vi "Launch.vi"() -> ()   [LabVIEW 2020]
uses:
  Supervision/Supervision/Supervision.lvclass
  D:/Projets/STEP AT/LUGE 2022.2/UIA_Demo/support/UI_Actor.lvlibp/UI_Actor/UI_Actor.lvclass
  D&Cs/SCHEMA_01/SCHEMA_01/SCHEMA_01.lvclass
  D&Cs/SCHEMA_02/SCHEMA_02/SCHEMA_02.lvclass
  D&Cs/SCHEMA_03/SCHEMA_03/SCHEMA_03.lvclass
  support/UI_Actor.lvlibp/UI_Actor/ctl_AR_Parameters.ctl
  support/UI_Actor.lvlibp/UI_Actor/ctl_AR_Mode.ctl
  support/UI_Actor.lvlibp/UI_Actor/UI_Actor.lvclass
  support/UI_Actor.lvlibp/UI_Actor Messages/UI_AutoRefresh Msg/UI_AutoRefresh Msg.lvclass
  support/Databox.lvlibp
panel:
  in  "T_0":dbl(slide)=6.037735849056604 scale=0.0..10.0
  # "UIA Demo"
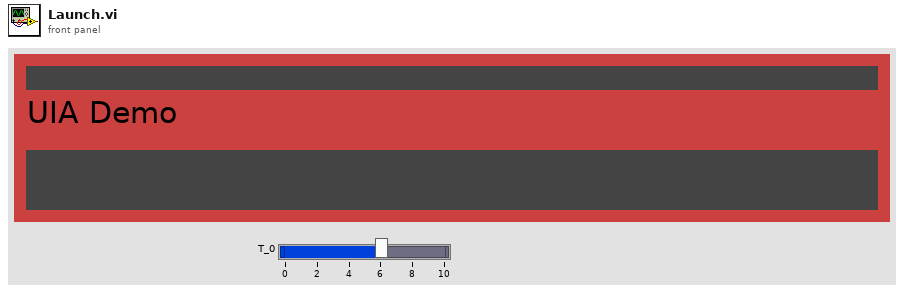
[diagram p1: front panel]
types:
  T1 = typedef "UI_Actor.lvlibp/UI_Actor.lvclass/ctl_AR_Parameters.ctl" = cluster{"Write TipStrips with details (T)":bool, "Write Captions with UserLabels (T)":bool, "Mode (ind only)":T2, "Enable nested stream (T)":bool}
  T2 = typedef "UI_Actor.lvlibp/UI_Actor.lvclass/ctl_AR_Mode.ctl" = enum16{"Controls only", "Indicators only", "All"}
  T3 = cluster{"Ch.Conf":refnum<class "Config.lvclass">, "Data":refnum<class "Data.lvclass">[]}
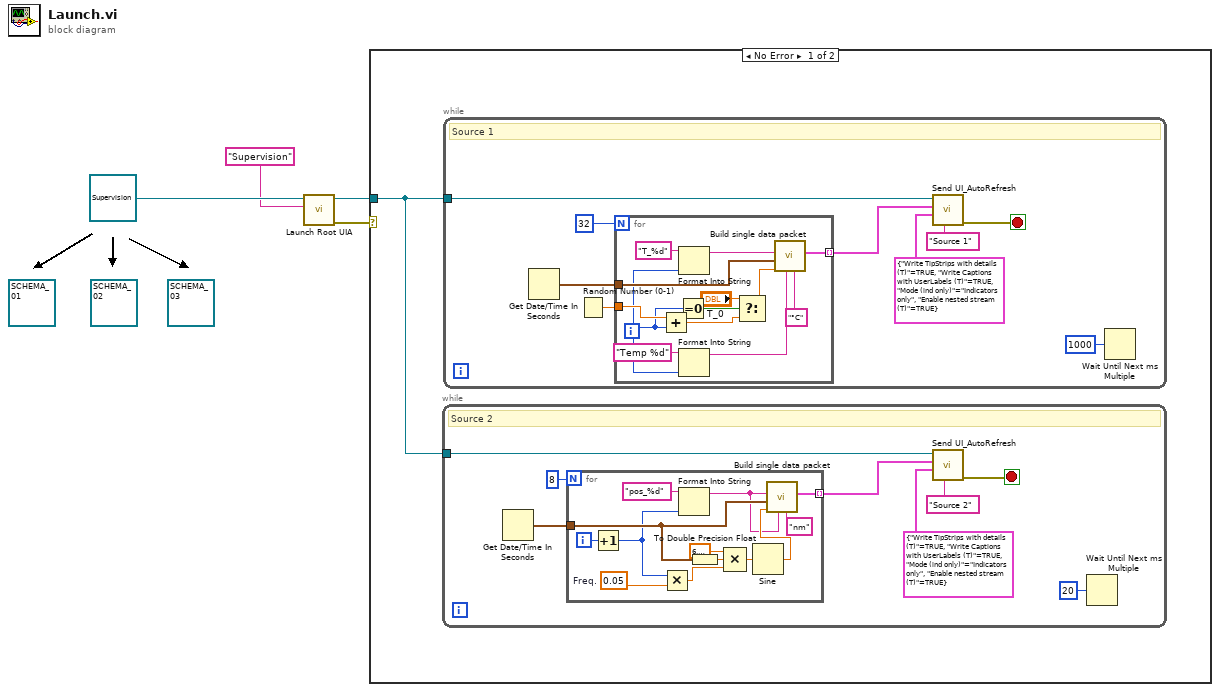
[diagram p0: block diagram]
diagram:
  (unwired) refnum<class "SCHEMA_03.lvclass"> refnum ("SCHEMA_03.lvlib:SCHEMA_03.lvclass")
  (unwired) refnum<class "SCHEMA_02.lvclass"> refnum ("SCHEMA_02.lvlib:SCHEMA_02.lvclass")
  (unwired) refnum<class "SCHEMA_01.lvclass"> refnum ("SCHEMA_01.lvlib:SCHEMA_01.lvclass")
  n1 = call "Launch Root UIA.vi"("Actor Name"="Supervision", "UI_Actor in"=refnum<class "Supervision.lvclass"> refnum ("LEF HMI.lvlib:LEF HMI.lvclass")) -> ("error out"=w1:errorcluster, "Actor's Enqueuer"=w2:refnum<class "Message Enqueuer.lvclass">)  [unwired: 8 in]
  n2 = case shown="No Error" w1 {
    tunnel: w2 -> [w5 _]
    frame No Error {
      n3 = while {
        tunnel: w5 -> [w34]
        stop <- w32 stop-if-true
        # "Source 2"
        n4 = Get Date/Time In Seconds() -> (seconds since 1Jan1904=w28:timestamp)
        n5 = for {
          N: 8 ("Nb aléa") -> [_]
          tunnel: [w47] -> w29 mode=indexing
          tunnel: w28 -> [w44]
          i -> [w41]
          w43 = 0.05  # Freq.
          n6 = Increment(x=w41) -> (x+1=w38:i32)
          n7 = Multiply(x=w38, y=w43) -> (x*y=w39:dbl)
          n8 = Format Into String(format string="pos_%d", w38) -> (resulting string=w37:string)  [unwired: 2 in, 1 out]
          n9 = To Double Precision Float(number=w44) -> (double precision float=w40:dbl)
          n10 = Compound Arithmetic op=MULTIPLY(6.283185307179586, w40, w39) -> (w46:dbl)
          n11 = Sine(x=w46) -> (sin(x)=w42:dbl)
          n12 = call "Build single data packet.vi"("Unit"="nm", "User Label"=w37, "Value"=w42, "Time (now!)"=w44, "System Label"=w37) -> ("DataPacket"=w47:T3)  [unwired: 6 in]
        }
        n13 = call "Send UI_AutoRefresh.vi"("Sourcer name"="Source 2" ("Sourcer 1"), "Parameters (Tipstrips,Captions,All)"=T1 {"Write TipStrips with details (T)"=TRUE, "Write Captions with UserLabels (T)"=TRUE, "Mode (ind only)"=enum."Indicators only", "Enable nested stream (T)"=TRUE}, "Data chunk"=w29, "Message Enqueuer"=w34) -> ("error out"=w32:errorcluster)  [unwired: 6 in, 1 out]
        n14 = Wait Until Next ms Multiple(millisecond multiple=u32 20) -> ()  [unwired: 1 out]
      }
      n15 = while {
        tunnel: w5 -> [w13]
        stop <- w6 stop-if-true
        # "Source 1"
        n16 = Get Date/Time In Seconds() -> (seconds since 1Jan1904=w7:timestamp)
        n17 = Random Number (0-1)() -> (number: 0 to 1=w11:dbl)
        n18 = for {
          N: 32 ("Nb aléa") -> [_]
          tunnel: [w25] -> w12 mode=indexing
          tunnel: w11 -> [w26]
          tunnel: w7 -> [w24]
          i -> [w17]
          n19 = Add(x=w26, y=w17) -> (x+y=w16:dbl)
          n20 = Equal To 0?(x=w17) -> (x = 0?=w19:bool)
          n21 = Format Into String(format string="T_%d", w17) -> (resulting string=w20:string)  [unwired: 2 in, 1 out]
          n22 = Format Into String(format string="Temp %d", w17) -> (resulting string=w22:string)  [unwired: 2 in, 1 out]
          n23 = Select(t="T_0", s=w19, f=w16) -> (s? t:f=w18:dbl)
          n24 = call "Build single data packet.vi"("Unit"="°C", "User Label"=w22, "Value"=w18, "Time (now!)"=w24, "System Label"=w20) -> ("DataPacket"=w25:T3)  [unwired: 6 in]
        }
        n25 = call "Send UI_AutoRefresh.vi"("Sourcer name"="Source 1" ("Sourcer 1"), "Parameters (Tipstrips,Captions,All)"=T1 {"Write TipStrips with details (T)"=TRUE, "Write Captions with UserLabels (T)"=TRUE, "Mode (ind only)"=enum."Indicators only", "Enable nested stream (T)"=TRUE}, "Data chunk"=w12, "Message Enqueuer"=w13) -> ("error out"=w6:errorcluster)  [unwired: 6 in, 1 out]
        n26 = Wait Until Next ms Multiple(millisecond multiple=u32 1000) -> ()  [unwired: 1 out]
      }
    }
    frame Error {
    }
  }
